vi "APS load sscnet servo abs position.vi"(7 "Res_Cnt":i32, 8 "error in (no error)":errorcluster caption="错误输入（无错误）", 9 "Cyc_Cnt":i32, 10 "Abs_Option":i32, 11 "Axis_ID":i32) -> (0 "error out":errorcluster caption="错误输出", 1 "Cyc_Cnt out":i32, 3 "function return":i32, 5 "Res_Cnt out":i32)   [LabVIEW 2011, in "APS168.lvlib"]
doc: "I32 FNTYPE APS_load_sscnet_servo_abs_position( I32 Axis_ID, I32 Abs_Option, I32 *Cyc_Cnt, I32 *Res_Cnt );"
uses:
  APS168.lvlib
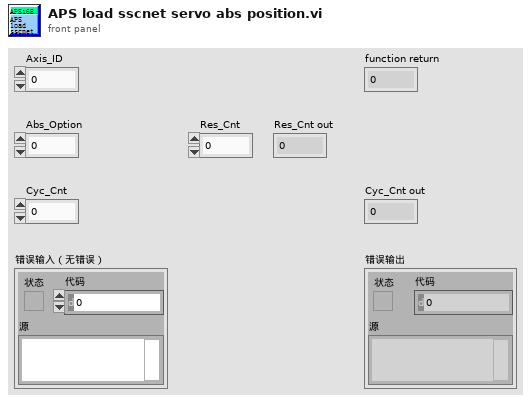
[diagram p1: front panel]
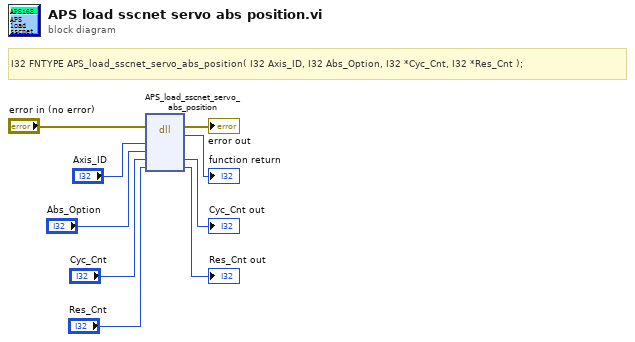
[diagram p0: block diagram]
diagram:
  # "I32 FNTYPE APS_load_sscnet_servo_abs_position( I32 Axis_ID, I32 Abs_Option, I32 *Cyc_Cnt, I32 *Res_Cnt );"
  n1 = dll-call lib="PTH1Labs E软件ADLINK 204CAPS_1_7_1_LIB line 连续运动204APS168.*" fn="APS_load_sscnet_servo_abs_position"(error in="error in (no error)", "Axis_ID"="Axis_ID", "Abs_Option"="Abs_Option", "Cyc_Cnt"="Cyc_Cnt", "Res_Cnt"="Res_Cnt") -> (error out=→"error out":errorcluster, →"function return":i32, "Cyc_Cnt"=→"Cyc_Cnt out":i32, "Res_Cnt"=→"Res_Cnt out":i32)  [unwired: 4 in, 1 out]
